vi "GUI_Bella_Laser_separate_graphs.vi"() -> ()   [LabVIEW 2013]
uses:
  shared programs/GUI_Template/GUI_master/tcp_new_data_event.ctl
  shared programs/GUI_Template/GUI_master/tcp new data cluster.ctl
panel:
  out "standard deviation 9":dbl caption="sigma" format="%.1f"
  out "mean 9":dbl caption="mean" format="%.1f"
  out "standard deviation 8":dbl caption="sigma" format="%.1f"
  out "mean 8":dbl caption="mean" format="%.1f"
  out "standard deviation 7":dbl caption="sigma" format="%.1f"
  out "mean 7":dbl caption="mean" format="%.1f"
  out "standard deviation 6":dbl caption="sigma" format="%.1f"
  out "mean 6":dbl caption="mean" format="%.1f"
  out "standard deviation 5":dbl caption="sigma" format="%.1f"
  out "mean 5":dbl caption="mean" format="%.1f"
  out "standard deviation 4":dbl caption="sigma" format="%.3f"
  out "standard deviation 3":dbl caption="sigma" format="%0.2f"
  out "standard deviation 2":dbl caption="sigma"
  out "standard deviation":dbl caption="sigma" format="%0.2f"
  in  "GUIdevice 4":string="LB_EnergyMeter_2"
  in  "GUIdevice 3":string="LB_EnergyMeter_1"
  out "mean 4":dbl caption="mean" format="%.3f"
  out "mean 3":dbl caption="mean" format="%0.2f"
  out "mean 2":dbl caption="mean"
  out "mean":dbl format="%.1f"
  out "XY Graph 8":cluster{dbl[], dbl[]}[](graph)
  out "XY Graph 7":cluster{dbl[], dbl[]}[](graph)
  out "XY Graph 6":cluster{dbl[], dbl[]}[](graph)
  out "XY Graph 5":cluster{dbl[], dbl[]}[](graph)
  out "XY Graph 4":cluster{dbl[], dbl[]}[](graph)
  out "XY Graph 3":cluster{dbl[], dbl[]}[](graph)
  out "XY Graph 2":cluster{dbl[], dbl[]}[](graph)
  out "XY Graph":cluster{dbl[], dbl[]}[](graph)
  in  "GUIdevice 2":string="RegenSpectrometer"
  out "FWHM::2":dbl caption="Regen FWHM" min=0.0 max=10000.0
  out "Thales.Spectrum_XPW_FWHM::1":dbl caption="Booster FWHM" min=-999.0 max=999999999.0
  out "Thales.Spectrum_Amp3_FWHM::1":dbl caption="Amp3 FWHM" min=-999.0 max=999999999.0
  out "Thales.Spectrum_Booster_FWHM::1":dbl caption="Booster FWHM" min=-999.0 max=999999999.0
  out "Thales.Spectrum_Preamp_FWHM::1":dbl caption="Amp1 FWHM" min=-999.0 max=999999999.0
  out "Thales.Spectrum_Regen_FWHM::1":dbl caption="Osc FWHM" min=-999.0 max=999999999.0
  in  "Clear":bool
  in  "GUIdevice 1":string="BELLA_ThalesSVE"
  out "Reading.Channel 2::4":dbl caption="Amp3 (J)" min=0.0 max=0.0 format="%#.3f"
  out "Reading.Channel 2::3":dbl caption="Amp1 (mJ)" min=0.0 max=0.0
  out "Reading.Channel 1::4":dbl caption="Amp2 (J)" min=0.0 max=0.0 format="%#.3f"
  out "Reading.Channel 1::3":dbl caption="Preamp (mJ)" min=0.0 max=0.0
  out "tcp data event":T1
  in  "stop":bool
  out "error IO 2":errorcluster
  # "BELLA LASER STATS"
  # "Target"
  # "Target"
  # "Target"
  # "Target"
  # "Target"
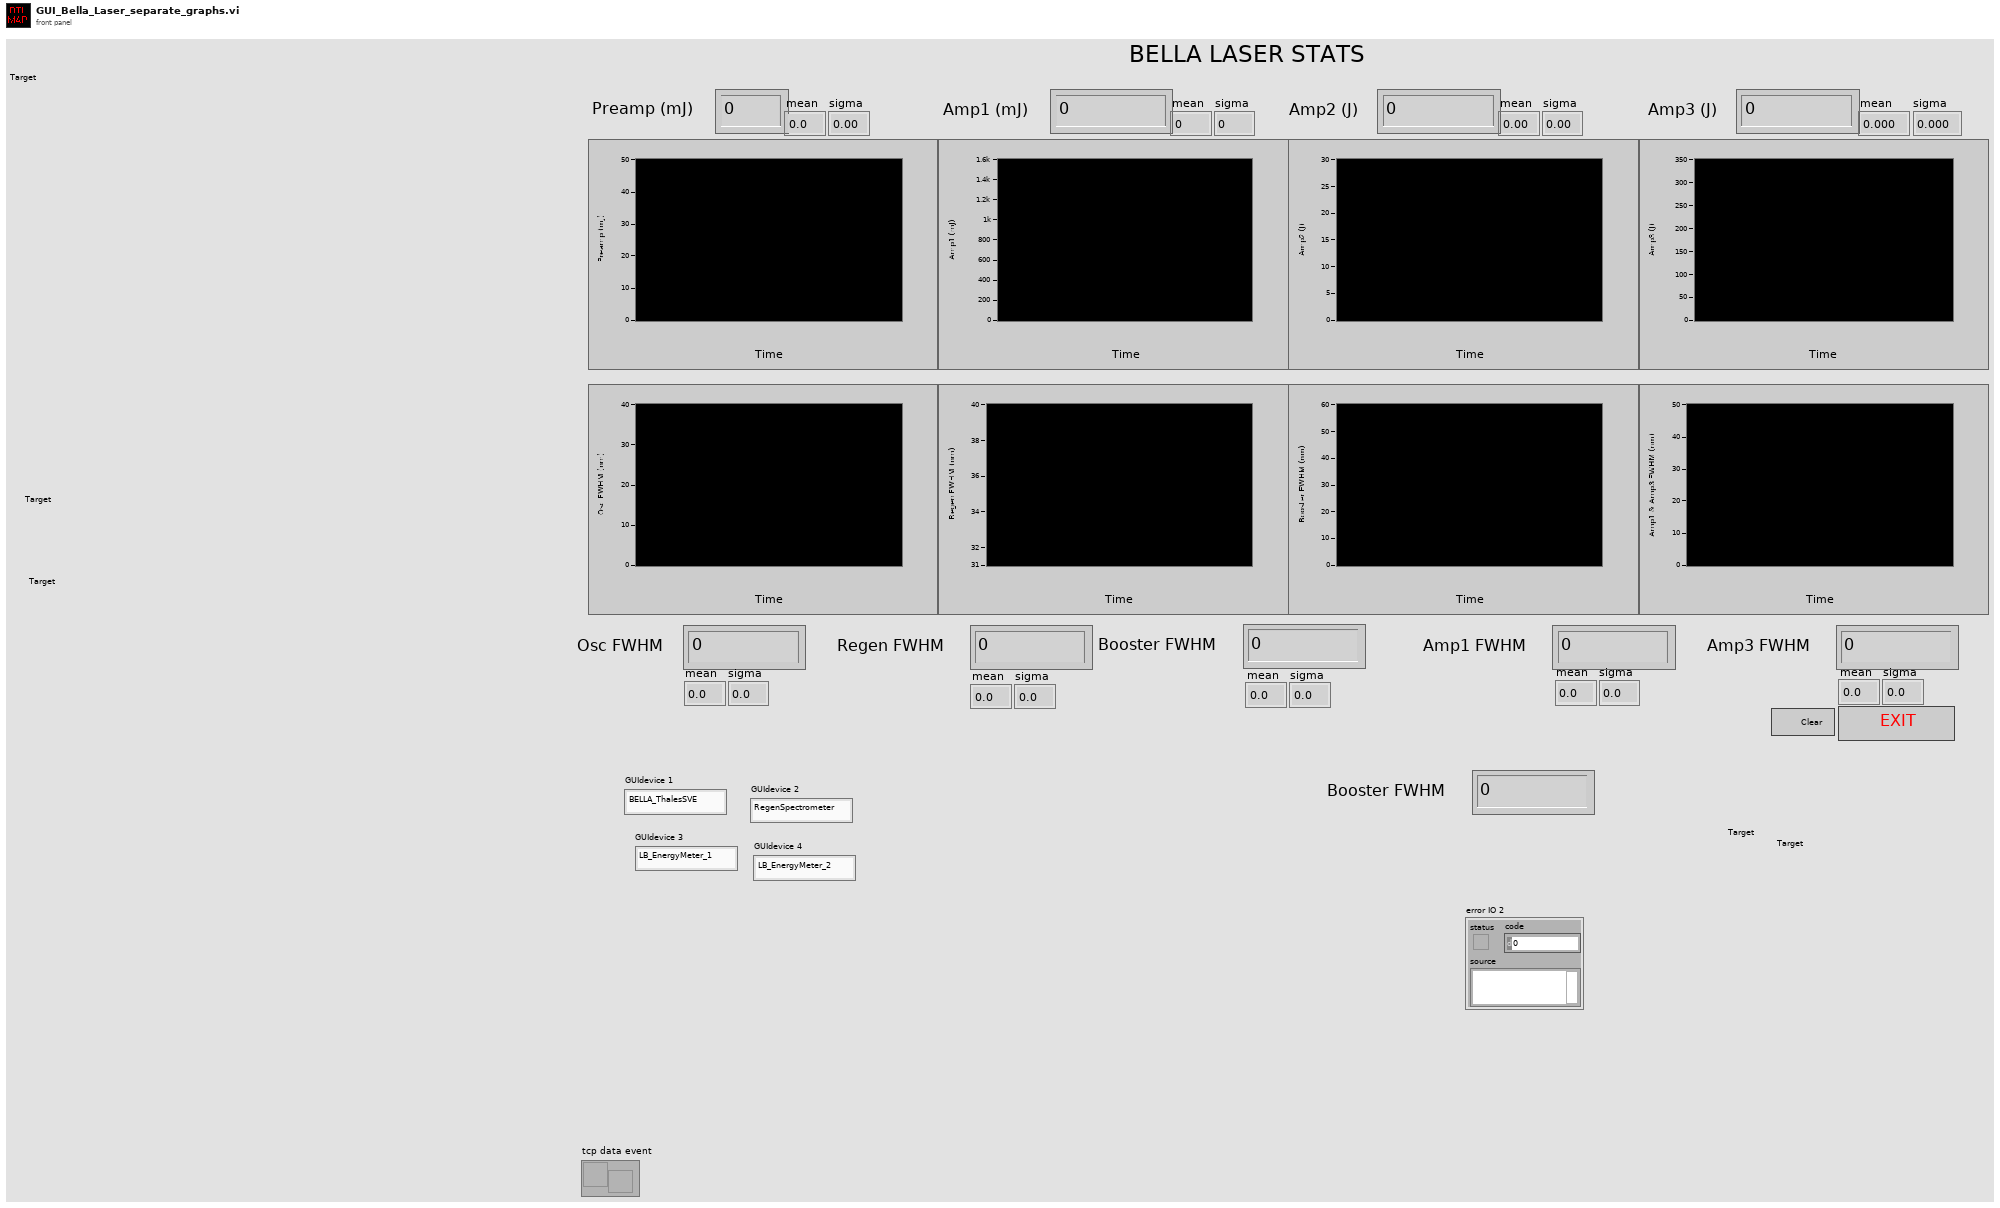
[diagram p1: front panel]
types:
  T1 = typedef "tcp_new_data_event.ctl" = refnum<user-event>
  T2 = typedef "tcp new data cluster.ctl" = cluster{"EventEnum":enum16{"new data", "connection status update"}, "Device name":string}
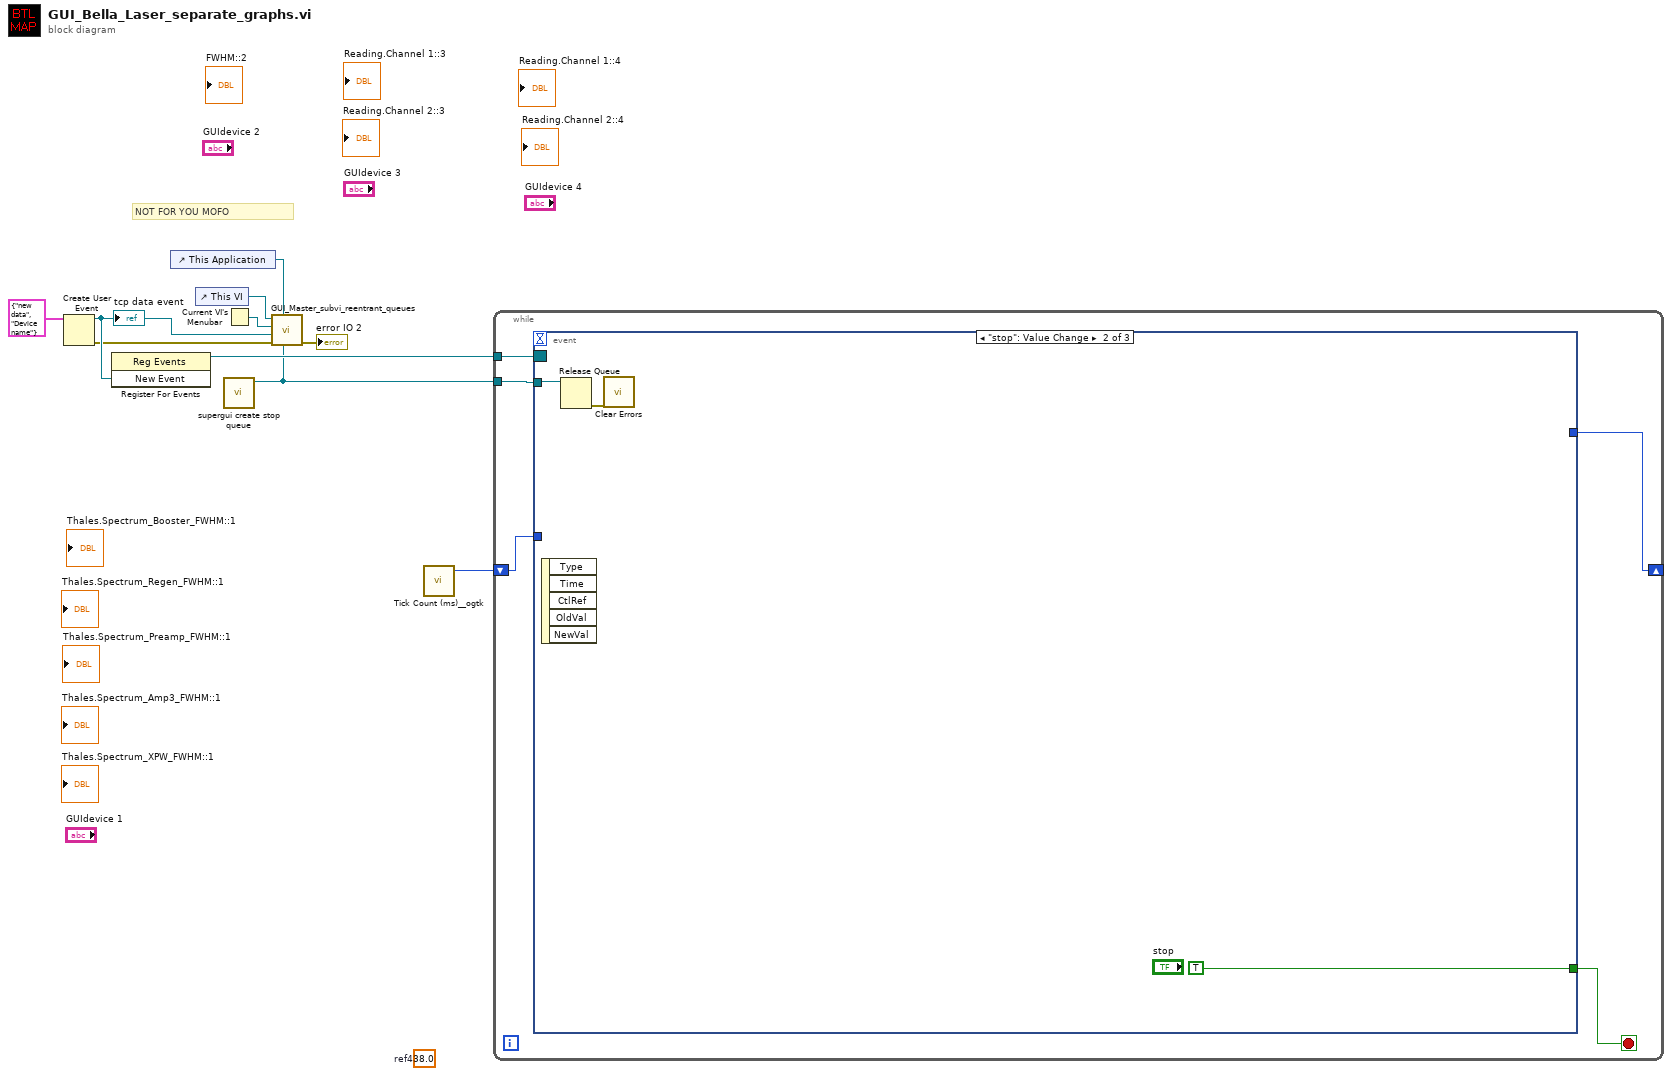
[diagram p0: block diagram]
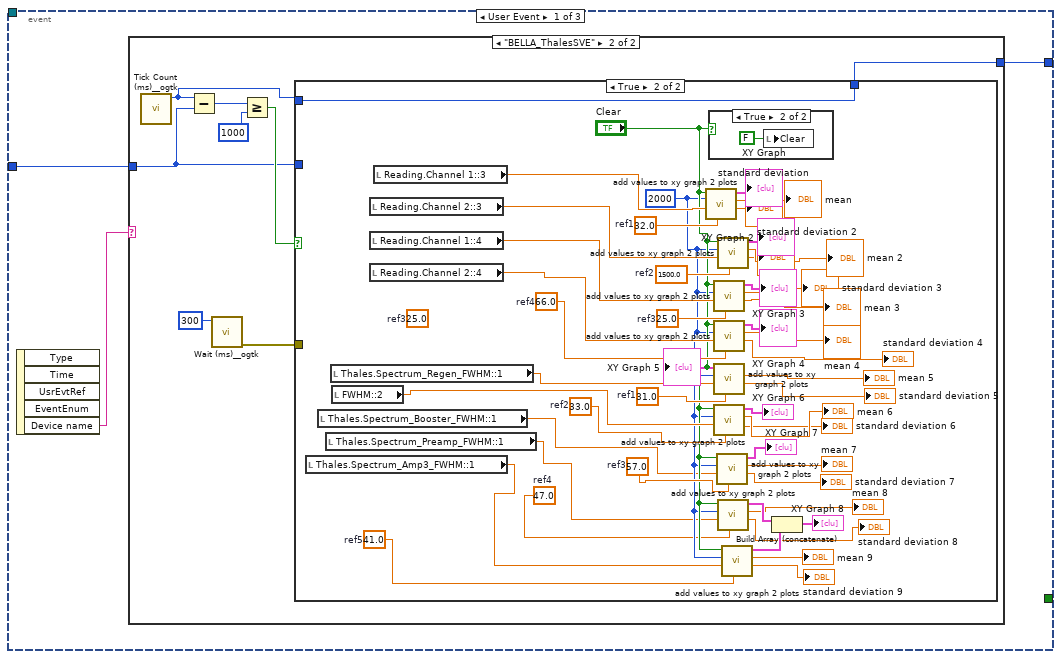
[diagram p2: hidden frame]
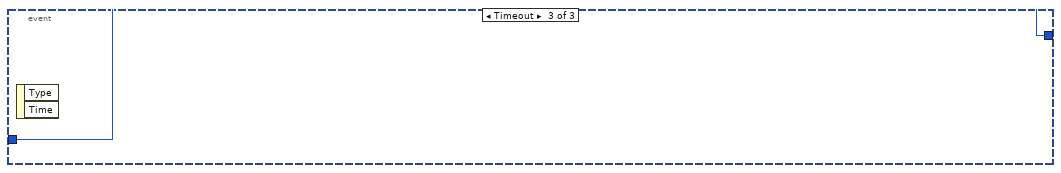
[diagram p6: hidden frame]
diagram:
  (unwired) 38.0  # ref4
  # "NOT FOR YOU MOFO"
  n1 = Create User Event(user event datatype=T2 {"EventEnum"=enum."new data", "Device name"="Device name"} ("New Event")) -> (user event=w9:refnum<user-event>, error out=w8:errorcluster)  [unwired: 1 in]
  "tcp data event" <- w9
  n2 = register-events(w9) -> (reference out=w4:refnum<event-registration>)  [unwired: 2 in, 1 out]
  n3 = control-ref of="This Application"() -> (w10:refnum<vi>)
  n4 = control-ref of="This VI"() -> (w5:refnum<vi>)
  n5 = call "supergui create stop queue.vi"() -> ("STOP Queue out"=w1:refnum<queue>)  [unwired: 11 in]
  n6 = Current VI's Menubar() -> (w6:refnum<k9>)
  n7 = call "GUI_Master_subvi_reentrant_queues.vi"("STOP Queue in"=w1, "This Application"=w10, "error in (no error)"=w8, "tcp data event"=w9, "Caller menu reference"=w6, "Caller VI ref"=w5) -> ("error out"=→"error IO 2":errorcluster)  [unwired: 5 in]
  n8 = call <userlib>:"Tick Count (ms)__ogtk.vi"() -> ("millisecond timer value"=w2:u32)  [unwired: 10 in, 1 out]
  n9 = while {
    tunnel: w4 -> [w14]
    shift-right: [w12] -> _
    shift-left: w2 -> [w13]
    tunnel: w1 -> [w11]
    stop <- w15 stop-if-true
    n10 = event shown="[1] \"stop\": Value Change" {
      selector: w14 -> [_ _ _]
      dyn-events: _ -> [_ _ _]
      timeout: _ -> [_ _ _]
      tunnel: [_ TRUE ("stop") _] -> w15
      tunnel: w13 -> [w17 _ w82]
      tunnel: [w16 _ w82] -> w12
      tunnel: w11 -> [_ w80 _]
      event User Event {
        n11 = event-data() -> ("Device name"=w18:string)  [unwired: 1 in, 4 out]
        n12 = case shown="\"BELLA_ThalesSVE\"" w18 {
          tunnel: w17 -> [w19 w24]
          tunnel: [w19 w22] -> w16
          frame Default {
          }
          frame "BELLA_ThalesSVE" {
            n13 = call <userlib>:"Tick Count (ms)__ogtk.vi"() -> ("millisecond timer value"=w23:u32)  [unwired: 10 in, 1 out]
            n14 = Subtract(x=w23, y=w24) -> (x-y=w26:u32)
            n15 = call <userlib>:"Wait (ms)__ogtk.vi"("milliseconds to wait"=u32 300) -> ("error out"=w21:errorcluster)  [unwired: 9 in, 1 out]
            n16 = Greater Or Equal?(x=w26, y=u32 1000 ("min time between updates")) -> (x >= y?=w25:bool)
            n17 = case shown="True" w25 {
              tunnel: w24 -> [w28 _]
              tunnel: w23 -> [_ w77]
              tunnel: [w28 w77] -> w22
              tunnel: w21 -> [_ _]
              frame False {
              }
              frame True {
                (unwired) 25.0  # ref3
                w48 = 41.0  # ref5
                w58 = 33.0  # ref2
                w50 = 47.0  # ref4
                w57 = 57.0  # ref3
                w60 = 31.0  # ref1
                w62 = 66.0  # ref4
                w67 = 25.0  # ref3
                w71 = 1500.0  # ref2
                w75 = 32.0  # ref1
                w52 = 2000 ("y")
                n18 = local read "Thales.Spectrum_Amp3_FWHM::1"() -> (w49:dbl)
                n19 = local read "Thales.Spectrum_Booster_FWHM::1"() -> (w43:dbl)
                n20 = local read "Thales.Spectrum_Preamp_FWHM::1"() -> (w51:dbl)
                n21 = local read "Thales.Spectrum_Regen_FWHM::1"() -> (w61:dbl)
                n22 = local read "FWHM::2"() -> (w59:dbl)
                n23 = local read "Reading.Channel 2::3"() -> (w72:dbl)
                n24 = local read "Reading.Channel 1::4"() -> (w70:dbl)
                n25 = local read "Reading.Channel 2::4"() -> (w66:dbl)
                n26 = local read "Reading.Channel 1::3"() -> (w76:dbl)
                n27 = call "add values to xy graph 2 plots.vi"("new value 2"=w75, "new value"=w76, "max # points"=w52, "Clear"="Clear") -> ("standard deviation"=→"standard deviation":dbl, "mean"=→"mean":dbl, "xy graph"=→"XY Graph":cluster{dbl[], dbl[]}[])  [unwired: 5 in]
                n28 = case shown="True" "Clear" {
                  frame False {
                  }
                  frame True {
                    n29 = local write "Clear"(FALSE ("Clear")) -> ()
                  }
                }
                n30 = call "add values to xy graph 2 plots.vi"("new value 2"=w67, "new value"=w70, "max # points"=w52, "Clear"="Clear") -> ("standard deviation"=→"standard deviation 3":dbl, "mean"=→"mean 3":dbl, "xy graph"=→"XY Graph 3":cluster{dbl[], dbl[]}[])  [unwired: 5 in]
                n31 = call "add values to xy graph 2 plots.vi"("new value 2"=w62, "new value"=w66, "max # points"=w52, "Clear"="Clear") -> ("standard deviation"=→"standard deviation 4":dbl, "mean"=→"mean 4":dbl, "xy graph"=→"XY Graph 4":cluster{dbl[], dbl[]}[])  [unwired: 5 in]
                n32 = call "add values to xy graph 2 plots.vi"("new value 2"=w60, "new value"=w61, "max # points"=w52, "Clear"="Clear") -> ("standard deviation"=→"standard deviation 5":dbl, "mean"=→"mean 5":dbl, "xy graph"=→"XY Graph 5":cluster{dbl[], dbl[]}[])  [unwired: 5 in]
                n33 = call "add values to xy graph 2 plots.vi"("new value 2"=w58, "new value"=w59, "max # points"=w52, "Clear"="Clear") -> ("standard deviation"=→"standard deviation 6":dbl, "mean"=→"mean 6":dbl, "xy graph"=→"XY Graph 6":cluster{dbl[], dbl[]}[])  [unwired: 5 in]
                n34 = call "add values to xy graph 2 plots.vi"("new value 2"=w57, "new value"=w43, "max # points"=w52, "Clear"="Clear") -> ("standard deviation"=→"standard deviation 7":dbl, "mean"=→"mean 7":dbl, "xy graph"=→"XY Graph 7":cluster{dbl[], dbl[]}[])  [unwired: 5 in]
                n35 = call "add values to xy graph 2 plots.vi"("new value 2"=w71, "new value"=w72, "max # points"=w52, "Clear"="Clear") -> ("standard deviation"=→"standard deviation 2":dbl, "mean"=→"mean 2":dbl, "xy graph"=→"XY Graph 2":cluster{dbl[], dbl[]}[])  [unwired: 5 in]
                n36 = call "add values to xy graph 2 plots.vi"("new value 2"=w50, "new value"=w51, "max # points"=w52, "Clear"="Clear") -> ("standard deviation"=→"standard deviation 8":dbl, "mean"=→"mean 8":dbl, "xy graph"=w56:cluster{dbl[], dbl[]}[])  [unwired: 5 in]
                n37 = call "add values to xy graph 2 plots.vi"("new value 2"=w48, "new value"=w49, "max # points"=w52, "Clear"="Clear") -> ("standard deviation"=→"standard deviation 9":dbl, "mean"=→"mean 9":dbl, "xy graph"=w55:cluster{dbl[], dbl[]}[])  [unwired: 5 in]
                n38 = Build Array (concatenate)(w56, w55) -> (→"XY Graph 8":cluster{dbl[], dbl[]}[])
              }
            }
          }
        }
      }
      event "stop": Value Change {
        n39 = event-data() -> ()  [unwired: 1 in, 5 out]
        n40 = Release Queue(queue=w80) -> (error out=w79:errorcluster)  [unwired: 2 in, 2 out]
        n41 = call <vilib>:"Clear Errors.vi"("error in (no error)"=w79) -> ()  [unwired: 6 in, 1 out]
      }
      event Timeout {
        n42 = event-data() -> ()  [unwired: 1 in, 2 out]
      }
    }
  }
